vi "Pre Build.vi"(6 "Top Level/Always Included VIs":path[](array[path]), 7 "Main Destination Path":path, 9 "Target Name":string, 10 "Build Specification Name":string, 11 "Project Path":path) -> (0 "error out":errorcluster)   [LabVIEW 2015]
uses:
  <vilib>/AppBuilder/AB_API_Simple/Build Specification Version.ctl
  <vilib>/AppBuilder/AB_API_Simple/Set Build Specification Version (path).vi
  <vilib>/AppBuilder/AB_API_Simple/NI_App_Builder_API.lvlib
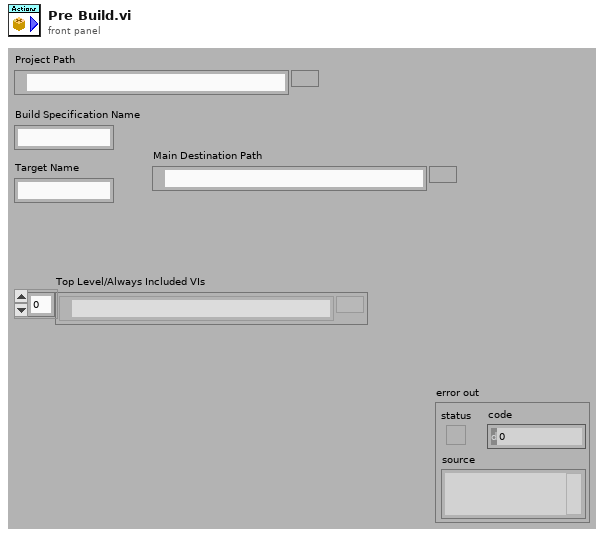
[diagram p1: front panel]
types:
  T1 = typedef "NI_App_Builder_API.lvlib/Build Specification Version.ctl" = cluster{"Major":u16, "Minor":u16, "Fix":u16, "Build":u16}
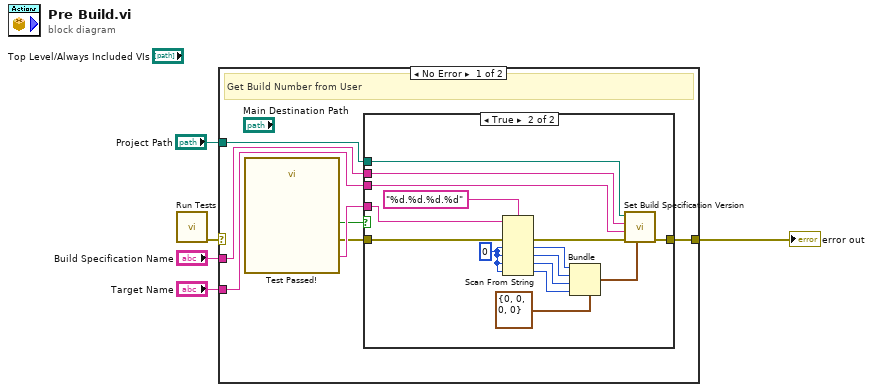
[diagram p0: block diagram]
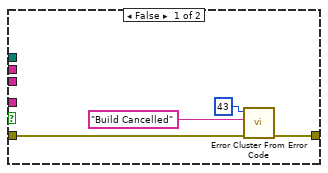
[diagram p2: hidden frame]
diagram:
  n1 = call "Run Tests.vi"() -> ("error out"=w5:errorcluster)  [unwired: 11 in]
  n2 = case shown="No Error" w5 {
    selector: w5 -> [_ w32]
    tunnel: [w9 w32] -> w1
    tunnel: "Project Path" -> [w8 _]
    tunnel: "Build Specification Name" -> [w7 _]
    tunnel: "Target Name" -> [w6 _]
    frame No Error {
      # "Get Build Number from User"
      n3 = call "Test Passed!"() -> ("Release Build"=w12:string, "OK"=w10:bool, "error out"=w11:errorcluster)  [unwired: 17 in]
      n4 = case shown="True" w10 {
        tunnel: w12 -> [_ w31]
        tunnel: w11 -> [w16 w28]
        tunnel: [w13 w17] -> w9
        tunnel: w8 -> [_ w27]
        tunnel: w7 -> [_ w19]
        tunnel: w6 -> [_ w18]
        frame False {
          n5 = call <vilib>:"Error Cluster From Error Code.vi"("error in (no error)"=w16, "error message (\"\")"="Build Cancelled" ("error message (\"\")"), "error code (0)"=43) -> ("error out"=w13:errorcluster)  [unwired: 6 in]
        }
        frame True {
          w29 = u16 0 ("default value 1")
          n6 = Scan From String(format string="%d.%d.%d.%d", input string=w31, error in=w28, default 1=w29, default 2=w29, default 3=w29, default 4=w29) -> (error out=w26:errorcluster, output 1=w23:u16, output 2=w22:u16, output 3=w21:u16, output 4=w20:u16)  [unwired: 1 in, 2 out]
          n7 = Bundle(cluster=T1 {"Major"=0, "Minor"=0, "Fix"=0, "Build"=0} ("Build Specification Version"), "Major"=w23, "Minor"=w22, "Fix"=w21, "Build"=w20) -> (w24:T1)
          n8 = call-poly <vilib>:"Set Build Specification Version.vi"("Build Specification Version"=w24, "error in (no error)"=w26, "Name of target (My Computer)"=w18, "Name of build specification"=w19, "Path to project"=w27) -> ("error out"=w17:errorcluster)  [unwired: 6 in]
        }
      }
    }
    frame Error {
    }
  }
  "error out" <- w1
